vi "测试-生成模板备份.vi"(11 "输入产品序号":string) -> (1 "new path":path, 2 "保存路径":path, 3 "模板路径":path, 4 "检查文件路径是否正确":bool caption="文件或文件夹存在？")   [LabVIEW 2018]
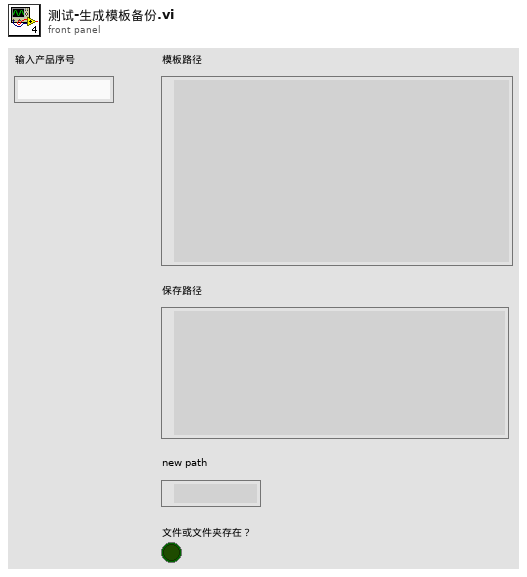
[diagram p1: front panel]
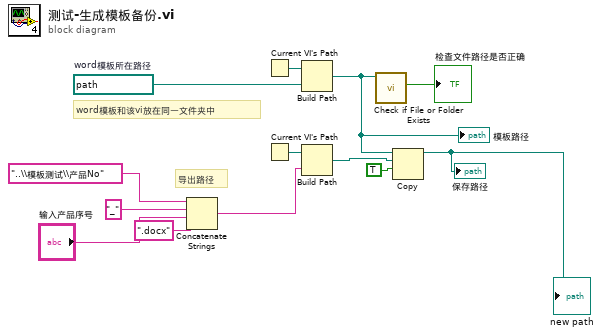
[diagram p0: block diagram]
diagram:
  w2 = path "../模板.docx"  # word模板所在路径
  # "导出路径"
  # "word模板和该vi放在同一文件夹中"
  n1 = Concatenate Strings("..\\模板测试\\产品No" ("字符串"), "_" ("名称或相对路径"), "输入产品序号", ".docx" ("名称或相对路径")) -> (w13:string)
  n2 = Current VI's Path() -> (path=w1:path)
  n3 = Current VI's Path() -> (path=w4:path)
  n4 = Build Path(base path=w1, name or relative path=w2) -> (appended path=w6:path)
  "模板路径" <- w6
  n5 = Build Path(base path=w4, name or relative path=w13) -> (appended path=w5:path)
  n6 = call <vilib>:"Check if File or Folder Exists.vi"("path"=w6) -> ("file or folder exists?"=→"检查文件路径是否正确":bool)  [unwired: 8 in, 2 out]
  n7 = Copy(9:TRUE ("覆盖(F)"), 10:w5, 11:w6) -> (3:→"保存路径" →"new path":path)  [unwired: 2 in, 2 out]
